vi "SwerveMapping.vi"(8 "Turn":dbl, 9 "Y Axis":dbl, 10 "X Axis":dbl, 11 "DriveIn":dbl) -> (3 "DriveOut":dbl)   [LabVIEW 2017]
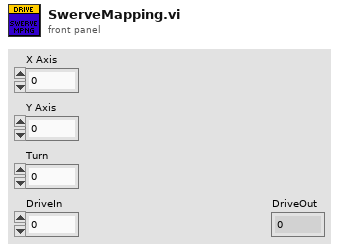
[diagram p1: front panel]
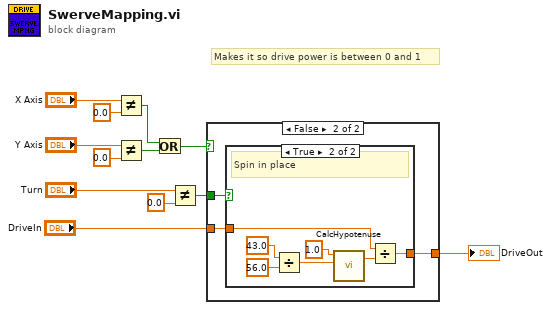
[diagram p0: block diagram]
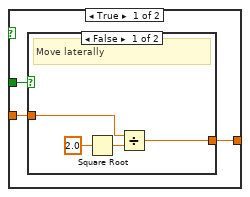
[diagram p2: hidden frame]
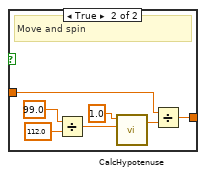
[diagram p3: hidden frame]
diagram:
  # "Makes it so drive power is between 0 and 1"
  n1 = Not Equal?(x="X Axis", y=0.0) -> (x != y?=w5:bool)
  n2 = Not Equal?(x="Y Axis", y=0.0) -> (x != y?=w4:bool)
  n3 = Or(x=w5, y=w4) -> (x .or. y?=w3:bool)
  n4 = Not Equal?(x="Turn", y=0.0) -> (x != y?=w2:bool)
  n5 = case shown="False" w3 {
    tunnel: "DriveIn" -> [w15 w28]
    tunnel: w2 -> [w13 w29]
    tunnel: [w14 w27] -> w1
    frame True {
      n6 = case shown="False" w13 {
        tunnel: w15 -> [w17 w21]
        tunnel: [w16 w20] -> w14
        frame False {
          # "Move laterally"
          n7 = Square Root(x=2.0) -> (sqrt(x)=w18:dbl)
          n8 = Divide(x=w17, y=w18) -> (x/y=w16:dbl)
        }
        frame True {
          # "Move and spin"
          n9 = Divide(x=99.0, y=112.0) -> (x/y=w26:dbl)
          n10 = call "CalcHypotenuse.vi"("b"=w26, "a"=1.0 ("x")) -> ("hypotenuse"=w22:dbl)  [unwired: 3 in]
          n11 = Divide(x=w21, y=w22) -> (x/y=w20:dbl)
        }
      }
    }
    frame False {
      n12 = case shown="True" w29 {
        tunnel: w28 -> [w30 w33]
        tunnel: [w30 w31] -> w27
        frame False {
          # "Not moving"
        }
        frame True {
          # "Spin in place"
          n13 = Divide(x=43.0, y=56.0) -> (x/y=w36:dbl)
          n14 = call "CalcHypotenuse.vi"("b"=w36, "a"=1.0 ("x")) -> ("hypotenuse"=w32:dbl)  [unwired: 3 in]
          n15 = Divide(x=w33, y=w32) -> (x/y=w31:dbl)
        }
      }
    }
  }
  "DriveOut" <- w1
